vi "GetWallError.vi"(8 "Lidar Magnitude":dbl[](array[numeric]), 11 "Target Distance":dbl) -> (0 "Errror":dbl, 3 "OH SHIT NO LIDAR DATA!!!":bool)   [LabVIEW 2016]
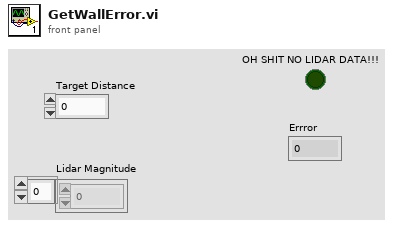
[diagram p1: front panel]
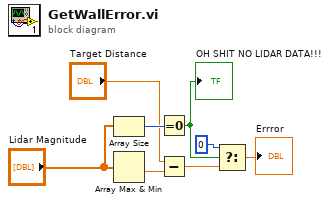
[diagram p0: block diagram]
diagram:
  n1 = Array Size(array="Lidar Magnitude") -> (size(s)=w8:i32)
  n2 = Array Max & Min(array="Lidar Magnitude") -> (min value=w6:dbl)  [unwired: 3 out]
  n3 = Equal To 0?(x=w8) -> (x = 0?=w4:bool)
  "OH SHIT NO LIDAR DATA!!!" <- w4
  n4 = Subtract(x="Target Distance", y=w6) -> (x-y=w2:dbl)
  n5 = Select(t=0, s=w4, f=w2) -> (s? t:f=→"Errror":dbl)
